vi "PH_ImageCoG_Plotter.PC Select Cam.vi"(0 "i ref in":refnum<vi>, 2 "Cam Instance":string="N/A", 5 "error in (no error)":errorcluster) -> (14 "i ref out":refnum<vi>, 19 "error out":errorcluster)   [LabVIEW 2014, in "PH_ImageCoG_Plotter.lvlib"]
uses:
  PH_ImageCoG_Plotter.lvlib
  PH_ImageCalibrator/PH_ImageCalibrator.lvlib
  PH_Img_BaseClass/PH_Img_BaseClass.lvlib
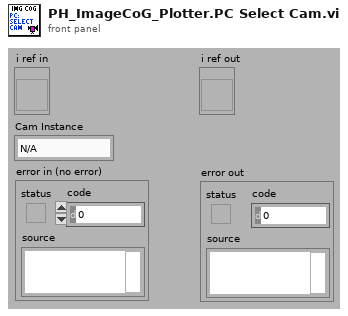
[diagram p1: front panel]
types:
  T1 = typedef "PH_Img_BaseClass.lvlib/PH_Img_BaseClass.i attribute.ctl" = cluster{"GUI Refs":T2, "Timeout Image [ms]":i32, "Default Periodic Period [ms]":i32, "Camera":cluster{"Instancename":string, "Notifier":refnum<notifier>}, "Palette":T3, "Cam Settings":cluster{"Cam ID":string, "Gain":dbl, "Brightness":dbl, "Shutter":dbl, "Cam Info Failure":bool, "Mode":i32}}
  T2 = typedef "PH_Img_BaseClass.lvlib/PH_Img_BaseClass.GUI Refs.ctl" = cluster{"Timeout":refnum<vi>, "Image":refnum<vi>, "Palette":refnum<vi>, "Timeout Set":refnum<vi>}
  T3 = typedef "PH_Img_BaseClass.lvlib/PH_Img_BaseClass.Palette.ctl" = i32
  T4 = typedef "PH_ImageCoG_Plotter.lvlib/PH_ImageCoG_Plotter.i attribute.ctl" = cluster{"GUI Refs":cluster{"Delete":refnum<vi>, "Calibration status":refnum<vi>, "BI subtracted":refnum<vi>, "calc Beam Anal":refnum<vi>, "CoG - x":refnum<vi>, "CoG - y":refnum<vi>, "Type":refnum<vi>, "Center":refnum<vi>, "exp - X":refnum<vi>, "exp - Y":refnum<vi>, "Delta - X":refnum<vi>, "Delta - Y":refnum<vi>, "Available Cams":refnum<vi>, "CoG X":refnum<vi>, "CoG Y":refnum<vi>, "Delta X":refnum<vi>, "Delta Y":refnum<vi>, "Export Data":refnum<vi>, "Calibration data":refnum<vi>}, "Calibration":cluster{"Status":T5, "Calibration data":T6, "Calibration Data File":path}, "Beam Analysis":cluster{"on":bool, "exp - X":i32, "exp - Y":i32, "Type":bool, "Data":cluster{"current time":timestamp, "CoG-x":dbl, "CoG-y":dbl, "Delta-x":dbl, "Delta-y":dbl}[], "Datasets strored":i32, "Dataarray Size":i32}, "Cam instances":string[], "DIM Service Events":T7[], "Images":cluster{"Background":T10, "OP":T10, "GUI":T10}}
  T5 = typedef "PH_StatusHandler.lvlib/PH_StatusHandler.Status.ctl" = i16
  T6 = typedef "PH_ImageCalibrator.lvlib/PH_ImageCalibrator.Calibration Data.ctl" = cluster{"Date":string, "Time":string, "Cam Settings":cluster{"Cam ID":string, "Gain":dbl, "Brightness":dbl, "Shutter":dbl, "Cam Error":bool, "Mode":i32}, "Background Image":cluster{"Image":dbl[][], "Image Error":bool}, "Linear Calibration":cluster{"Calibration Factor":dbl, "not mm or mrad":bool}, "Energy Calibration":cluster{"Calibration Factor":dbl, "no mJ":bool}}
  T7 = typedef "BaseProcess.lvlib/BaseProcess.event definition.ctl" = cluster{"CAEEvtDef":T8, "Data Descriptor":T9}
  T8 = typedef "CAEObj.lvlib/CAEObj.event definition.ctl" = cluster{"URL":string, "enable":bool, "ignoreResID":bool}
  T9 = typedef "BaseProcess.lvlib/BaseProcess.descriptor string definition.ctl" = string
  T10 = typedef "IMAQ Image.ctl" = refnum<image>
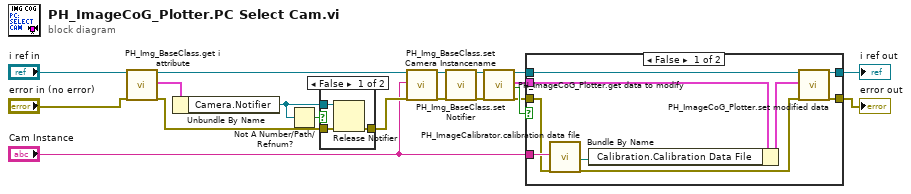
[diagram p0: block diagram]
diagram:
  n1 = call "PH_Img_BaseClass.get i attribute.vi"("i ref in"="i ref in", "error in (no error)"="error in (no error)") -> ("i ref out"=w11:refnum<vi>, "i attribute"=w10:T1, "error out"=w9:errorcluster)  [unwired: 15 in]
  n2 = Unbundle By Name(w10) -> ("Camera.Notifier"=w7:refnum<notifier>)
  n3 = Not A Number/Path/Refnum?(number/path/refnum=w7) -> (NaN/Path/Refnum?=w6:bool)
  n4 = case shown="False" w6 {
    tunnel: w9 -> [w22 w23]
    tunnel: [w21 w23] -> w8
    tunnel: w7 -> [w20 _]
    frame False {
      n5 = Release Notifier(notifier=w20, error in (no error)=w22) -> (error out=w21:errorcluster)  [unwired: 1 in, 2 out]
    }
    frame True {
    }
  }
  n6 = call "PH_Img_BaseClass.set Camera Instancename.vi"("i ref in"=w11, "Camera Instancename"="Cam Instance", "error in (no error)"=w8) -> ("i ref out"=w4:refnum<vi>, "error out"=w2:errorcluster)  [unwired: 15 in]
  n7 = call "PH_Img_BaseClass.set Notifier.vi"("i ref in"=w4, "error in"=w2) -> ("i ref out"=w3:refnum<vi>, "error out"=w1:errorcluster)  [unwired: 16 in]
  n8 = call "PH_ImageCoG_Plotter.get data to modify.vi"("i ref in"=w3, "error in (no error)"=w1) -> ("i ref out"=w14:refnum<vi>, "i attribute"=w16:T4, "timed out"=w15:bool, "error out"=w13:errorcluster)  [unwired: 14 in]
  n9 = case shown="False" w15 {
    tunnel: w13 -> [w24 w33]
    tunnel: [w32 w33] -> w18
    tunnel: [w31 w34] -> w19
    tunnel: w14 -> [w30 w34]
    tunnel: w16 -> [w28 _]
    tunnel: "Cam Instance" -> [w27 _]
    frame False {
      n10 = call "PH_ImageCalibrator.calibration data file.vi"("Camera Instance"=w27, "error in"=w24) -> ("File to save Cam Calibration Data in"=w26:path, "error out"=w25:errorcluster)  [unwired: 16 in]
      n11 = Bundle By Name(cluster=w28, "Calibration.Calibration Data File"=w26) -> (w29:T4)
      n12 = call "PH_ImageCoG_Plotter.set modified data.vi"("i ref in"=w30, "i attribute"=w29, "error in (no error)"=w25) -> ("i ref out"=w31:refnum<vi>, "error out"=w32:errorcluster)  [unwired: 15 in]
    }
    frame True {
    }
  }
  "i ref out" <- w19
  "error out" <- w18
